vi "LabVIEW IV 1주차.vi"() -> ()   [LabVIEW 2015]
uses:
  <vilib>/Analysis/1siggen.llb/Ramp Pattern by Samples.vi
  <vilib>/Analysis/NI_AALBase.lvlib
panel:
  in  "stop":bool
  in  "samples":i32=128
  in  "Voltage End":dbl
  in  "Voltage start":dbl
  out "XY Graph":cluster{"Y":dbl[], "Y":dbl[]}[](graph)
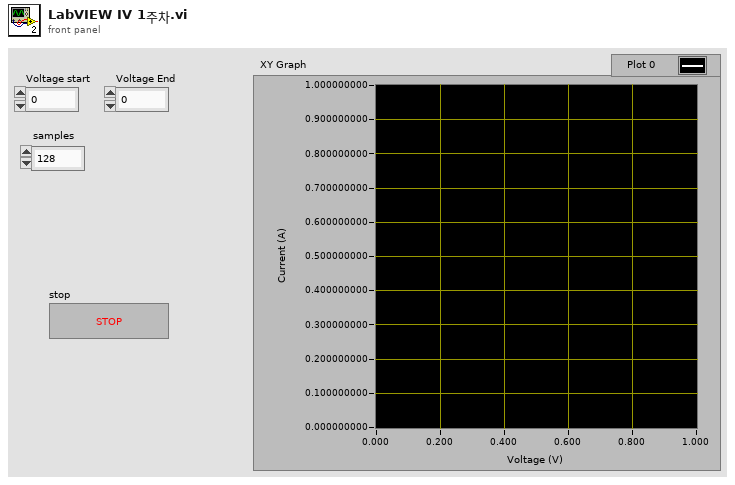
[diagram p1: front panel]
types:
  T1 = enum16{"open", "replace", "create", "open or create", "replace or create", "replace or create with confirmation"}
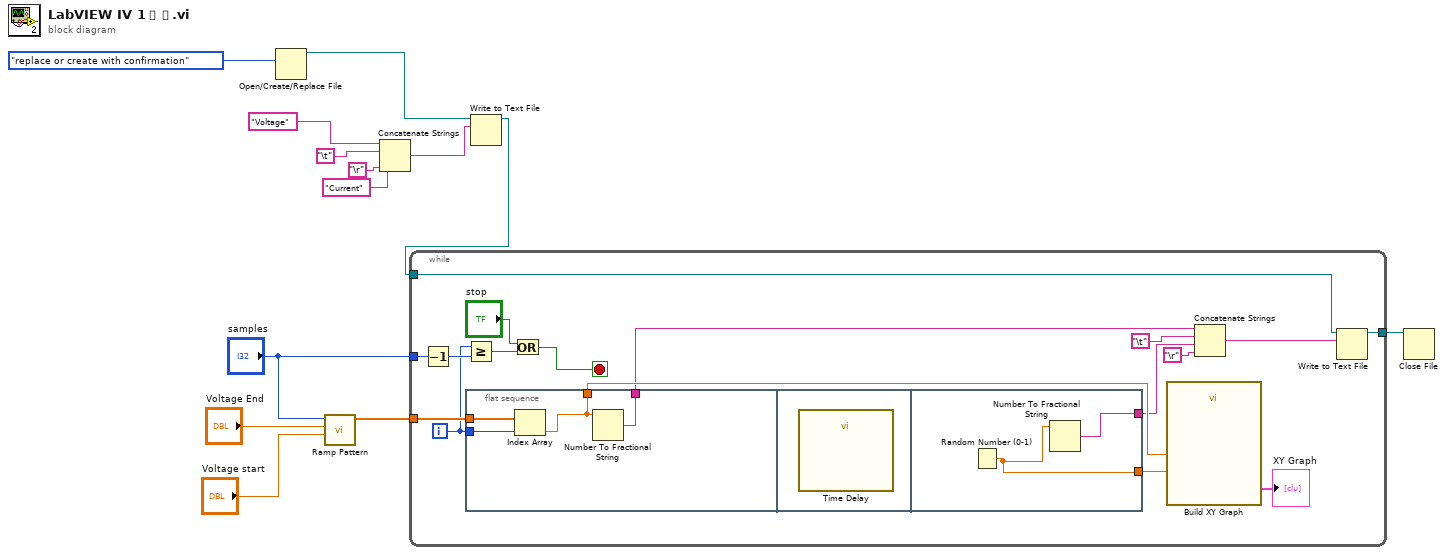
[diagram p0: block diagram]
diagram:
  n1 = Open/Create/Replace File(operation (0:open)=T1."replace or create with confirmation") -> (refnum out=w7:refnum<file>)  [unwired: 5 in, 2 out]
  n2 = call-poly <vilib>:"Ramp Pattern.vi"("start"="Voltage start", "end"="Voltage End", "samples"="samples") -> ("Ramp Pattern"=w11:dbl[])  [unwired: 7 in, 1 out]
  n3 = Concatenate Strings("Voltage" ("string"), "\t", "Current" ("string"), "\r") -> (w4:string)
  n4 = Write to Text File(file (use dialog)=w7, text=w4) -> (refnum out=w1:refnum<file>)  [unwired: 2 in, 2 out]
  n5 = while {
    tunnel: w11 -> [w30]
    tunnel: "samples" -> [w26]
    tunnel: w1 -> [w20]
    tunnel: [w19] -> w9
    i -> [w21]
    stop <- w22 stop-if-true
    n6 = Decrement(x=w26) -> (x-1=w25:i32)
    n7 = Greater Or Equal?(x=w21, y=w25) -> (x >= y?=w23:bool)
    n8 = flat-sequence {
      tunnel: w30 -> [w34]
      tunnel: w21 -> [w33]
      tunnel: [w32] -> w27
      tunnel: [w31] -> w18
      tunnel: [w36] -> w28
      tunnel: [w35] -> w17
      frame #0 {
        n9 = Index Array(array=w34, index=w33) -> (element=w32:dbl)
        n10 = Number To Fractional String(number=w32) -> (F-format string=w31:string)  [unwired: 3 in]
      }
      frame #1 {
        n11 = call "Time Delay"() -> ()  [unwired: 11 in, 1 out]
      }
      frame #2 {
        n12 = Random Number (0-1)() -> (number: 0 to 1=w36:dbl)
        n13 = Number To Fractional String(number=w36) -> (F-format string=w35:string)  [unwired: 3 in]
      }
    }
    n14 = Or(x="stop", y=w23) -> (x .or. y?=w22:bool)
    n15 = call "Build XY Graph"("Y Input"=w28, "X Input"=w27) -> ("XY Graph"=→"XY Graph":cluster{"X":dbl[], "Y":dbl[]}[])  [unwired: 8 in, 1 out]
    n16 = Concatenate Strings(w18, "\t", w17, "\r") -> (w14:string)
    n17 = Write to Text File(file (use dialog)=w20, text=w14) -> (refnum out=w19:refnum<file>)  [unwired: 2 in, 2 out]
  }
  n18 = Close File(refnum=w9) -> ()  [unwired: 1 in, 2 out]
